vi "Climber_Sequencer.vi"() -> (0 "Outer_Arm_Elevator":dbl, 1 "Inner_Arm_Pivot":dbl, 2 "Outer_Arm_Pivot":dbl)   [LabVIEW 2020]
panel:
  in  "Inner_Arm_Pivot_No_Load":T1={"Kp"=0.1, "Ki"=0.1, "Kd"=0.1, "N-Diff"=10, "N-Int"=20, "Int Error Window"=0.5, "Max Ouput"=1.0, "Min Output"=-1.0} {"Int Error Window" min=0.0; "N-Int" min=2; "N-Diff" min=2; "Kd" min=0.0; "Ki" min=0.0; "Kp" min=0.0}
  in  "Outer_Arm_Pivot_On_Bar":T1={"Kp"=0.1, "Ki"=0.1, "Kd"=0.1, "N-Diff"=10, "N-Int"=20, "Int Error Window"=0.5, "Max Ouput"=1.0, "Min Output"=-1.0} {"Int Error Window" min=0.0; "N-Int" min=2; "N-Diff" min=2; "Kd" min=0.0; "Ki" min=0.0; "Kp" min=0.0}
  in  "Outer_Arm_Pivot_No_Load":T1={"Kp"=0.1, "Ki"=0.1, "Kd"=0.1, "N-Diff"=10, "N-Int"=20, "Int Error Window"=0.5, "Max Ouput"=1.0, "Min Output"=-1.0} {"Int Error Window" min=0.0; "N-Int" min=2; "N-Diff" min=2; "Kd" min=0.0; "Ki" min=0.0; "Kp" min=0.0}
  in  "Outer_Elevator_No_Load":T1={"Kp"=0.1, "Ki"=0.1, "Kd"=0.1, "N-Diff"=10, "N-Int"=20, "Int Error Window"=0.5, "Max Ouput"=1.0, "Min Output"=-1.0} {"Int Error Window" min=0.0; "N-Int" min=2; "N-Diff" min=2; "Kd" min=0.0; "Ki" min=0.0; "Kp" min=0.0}
  in  "Outer_Elevator_On_Bar":T1={"Kp"=0.1, "Ki"=0.1, "Kd"=0.1, "N-Diff"=10, "N-Int"=20, "Int Error Window"=0.5, "Max Ouput"=1.0, "Min Output"=-1.0} {"Int Error Window" min=0.0; "N-Int" min=2; "N-Diff" min=2; "Kd" min=0.0; "Ki" min=0.0; "Kp" min=0.0}
  in  "No PID":T1={"Kp"=0.1, "Ki"=0.1, "Kd"=0.1, "N-Diff"=10, "N-Int"=20, "Int Error Window"=0.5, "Max Ouput"=1.0, "Min Output"=-1.0} {"Int Error Window" min=0.0; "N-Int" min=2; "N-Diff" min=2; "Kd" min=0.0; "Ki" min=0.0; "Kp" min=0.0}
  in  "step 7 phi0 error leniency":dbl
  in  "d4":dbl
  in  "phi2 error leniency":dbl
  in  "phi2":dbl
  in  "d3":dbl
  in  "phi1 error leniency":dbl
  in  "phi1":dbl
  in  "d2":dbl
  in  "phi0":dbl=90.0 format="%#_13g"
  in  "theta1":dbl
  in  "theta0":dbl
  in  "move step back":bool
  in  "confirm step advance":bool
  in  "reset":bool
  in  "inner_arm_rotation":dbl
  in  "outer_arm_rotation":dbl
  in  "d1":dbl
  in  "outer_arm_position":dbl
  out "step":i32
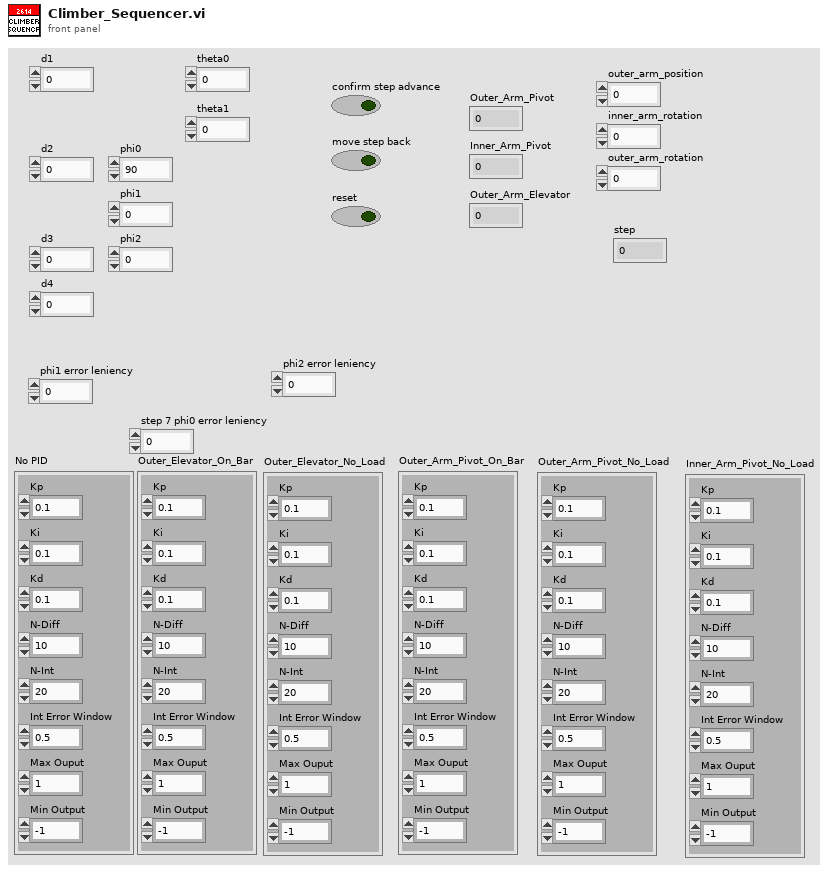
[diagram p1: front panel]
types:
  T1 = cluster{"Kp":dbl, "Ki":dbl, "Kd":dbl, "N-Diff":i32, "N-Int":i32, "Int Error Window":dbl, "Max Ouput":dbl, "Min Output":dbl}
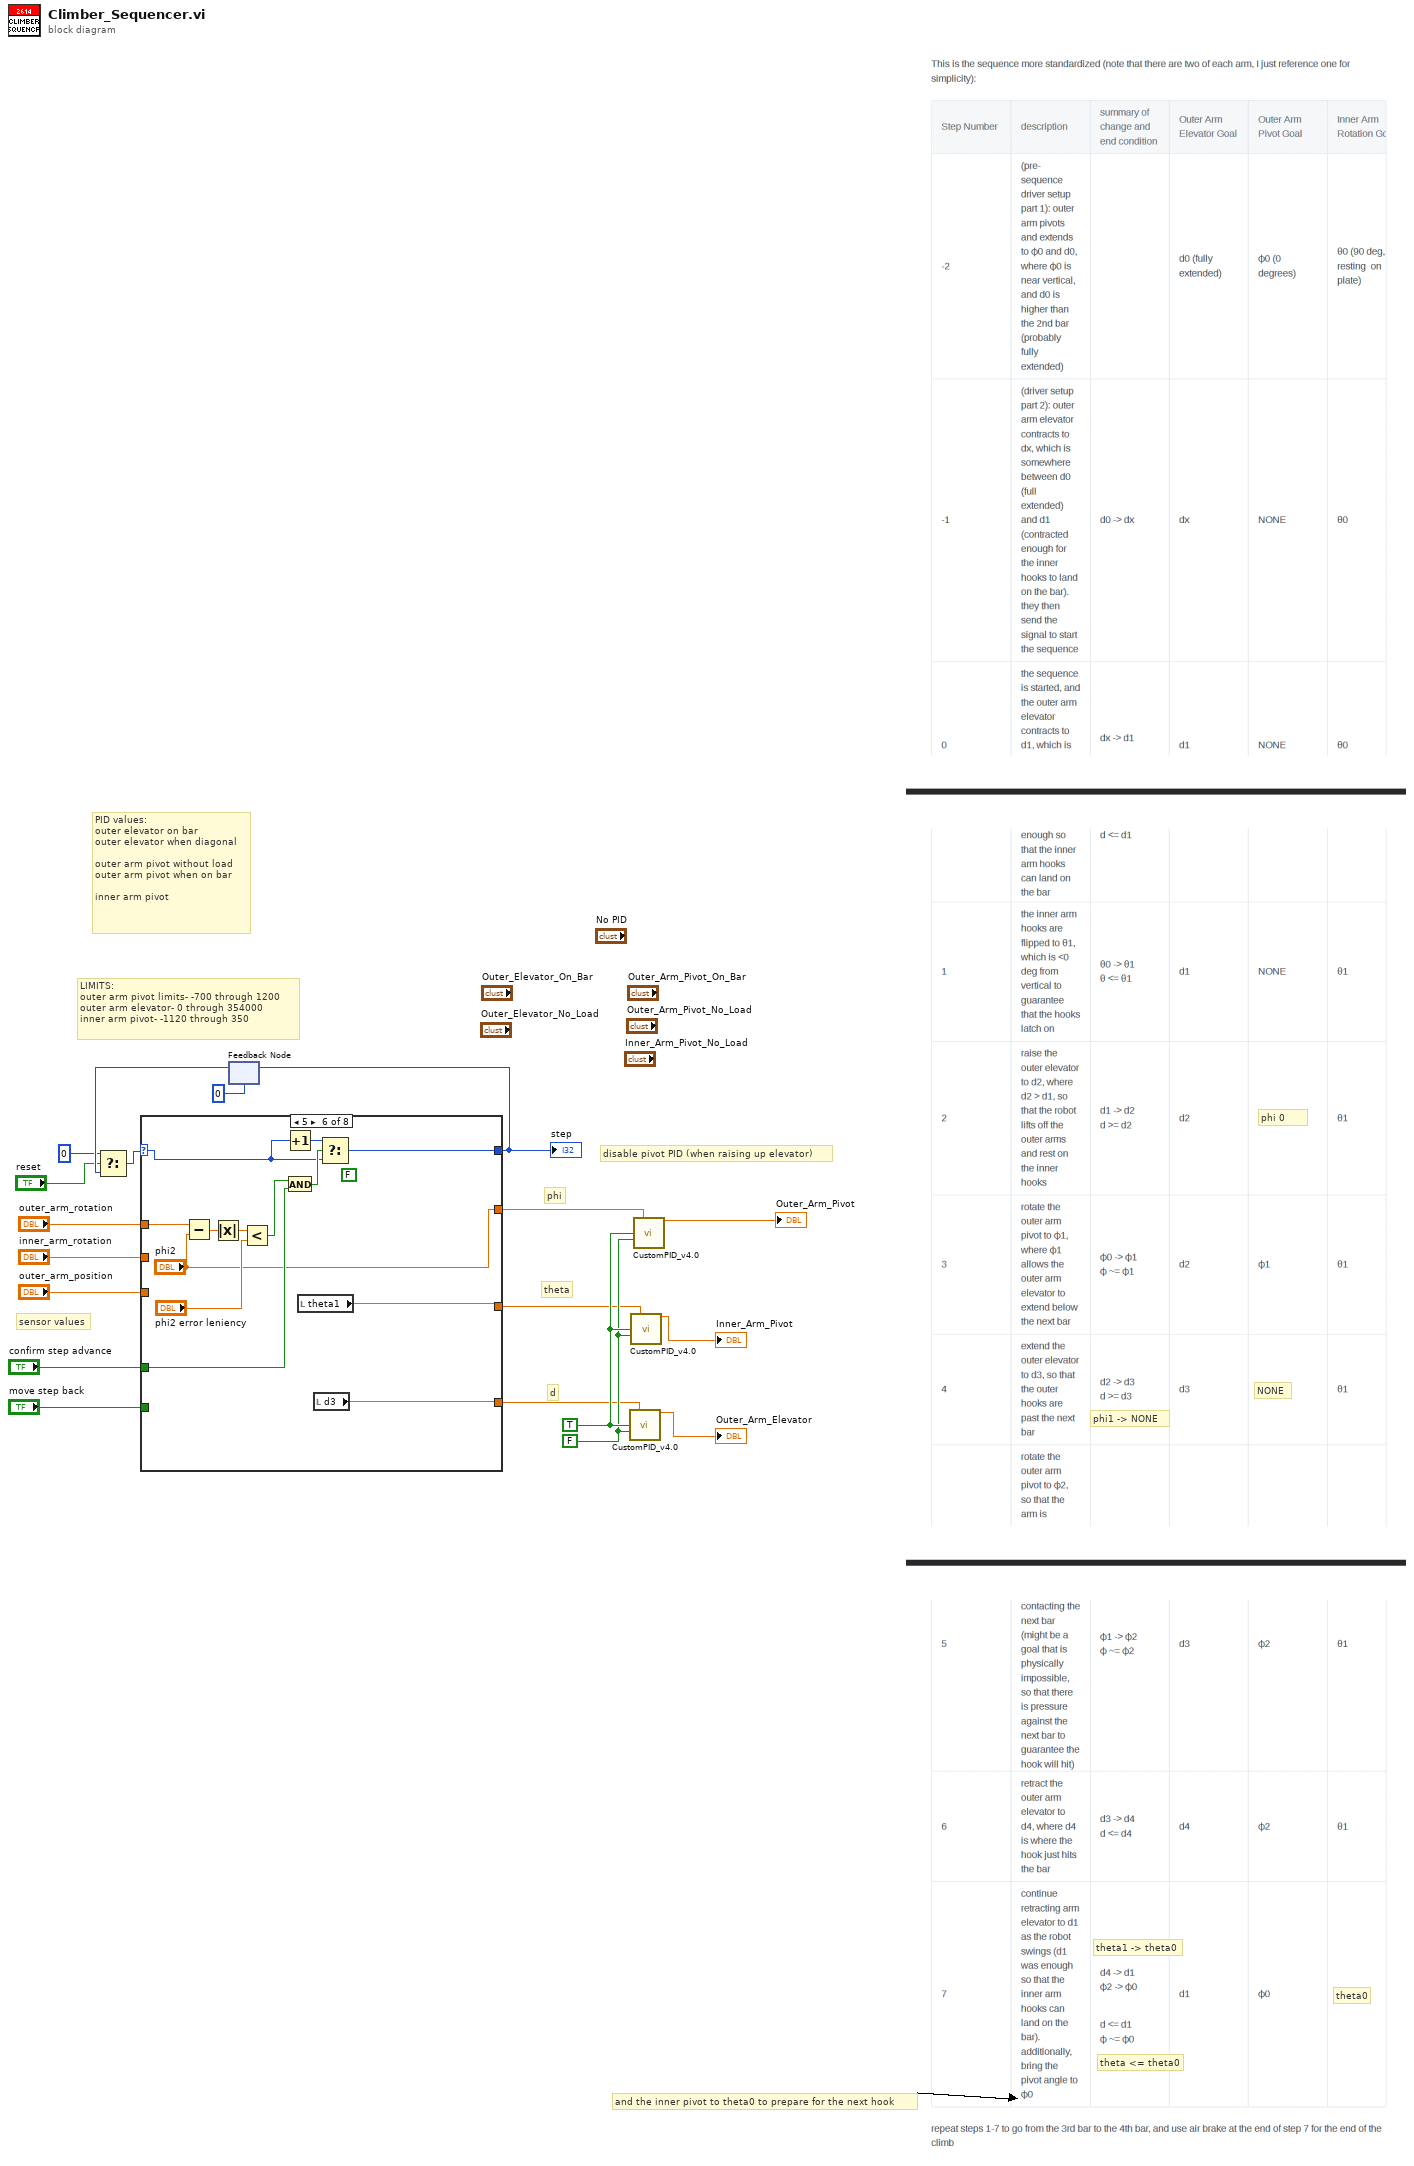
[diagram p0: block diagram]
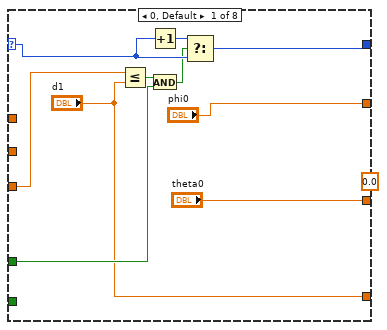
[diagram p2: hidden frame]
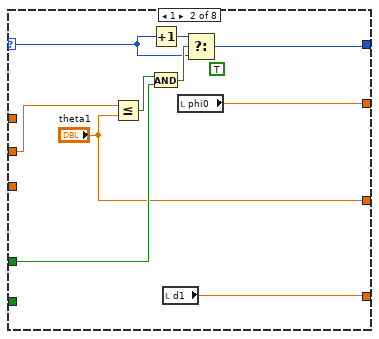
[diagram p3: hidden frame]
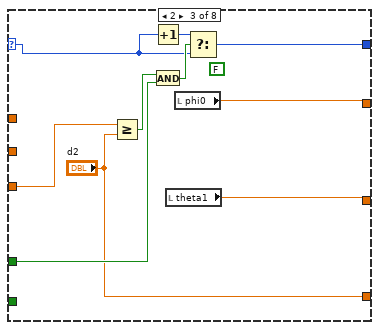
[diagram p4: hidden frame]
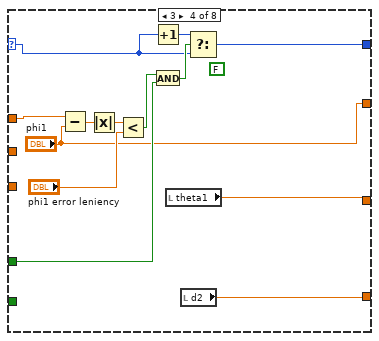
[diagram p5: hidden frame]
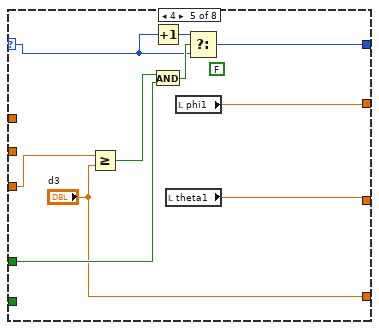
[diagram p6: hidden frame]
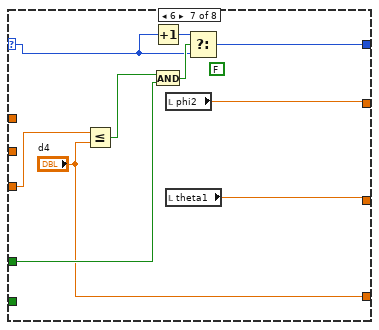
[diagram p7: hidden frame]
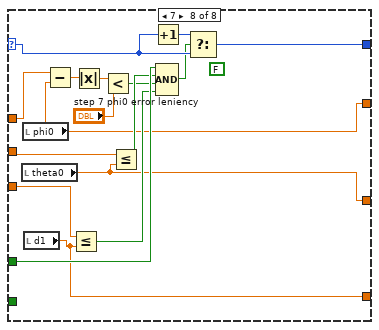
[diagram p8: hidden frame]
diagram:
  w9 = FALSE ("Reset on Goal Change ?")
  w10 = TRUE ("Reset on Goal Change ?")
  # "PID values:\nouter elevator on bar\nouter elevator when diagonal\n\nouter arm pivot without load\nouter arm pivot when on bar\n\ninner arm pivot"
  # "LIMITS:\nouter arm pivot limits- -700 through 1200\nouter arm elevator- 0 through 354000\ninner arm pivot- -1120 through 350"
  # "NONE"
  # "phi1 -> NONE"
  # "theta0"
  # "theta <= theta0"
  # "theta1 -> theta0"
  # "and the inner pivot to theta0 to prepare for the next hook"
  # "phi 0"
  # "disable pivot PID (when raising up elevator)"
  # "theta"
  # "phi"
  # "d"
  # "sensor values"
  n1 = feedback #1(0) -> (w16:i32)
  n2 = Select(t=0, s="reset", f=w16) -> (s? t:f=w17:i32)
  n3 = case shown="5" w17 {
    selector: w17 -> [w28 w36 w47 w60 w70 w83 w93 w111]
    tunnel: [w29 w37 w46 w59 w69 w82 w92 w110] -> w19
    tunnel: "outer_arm_position" -> [w26 _ w42 _ w65 _ w88 w107]
    tunnel: "confirm step advance" -> [w23 w35 w45 w58 w68 w81 w91 w108]
    tunnel: "move step back" -> [_ _ _ _ _ _ _ _]
    tunnel: ["phi0" w30 w44 "phi1" w66 "phi2" w89 w96] -> w6
    tunnel: "outer_arm_rotation" -> [_ _ _ w55 _ w77 _ w101]
    tunnel: "inner_arm_rotation" -> [_ w34 _ _ _ _ _ w103]
    tunnel: ["theta0" "theta1" w43 w57 w67 w80 w90 w102] -> w3
    tunnel: ["d1" w31 "d2" w56 "d3" w74 "d4" w105] -> w2
    frame 0, Default {
      (unwired) 0.0 ("d1")
      (unwired) 0.0 ("d1")
      n4 = Less Or Equal?(x=w26, y="d1") -> (x <= y?=w25:bool)
      n5 = Increment(x=w28) -> (x+1=w27:i32)
      n6 = And(x=w25, y=w23) -> (x .and. y?=w24:bool)
      n7 = Select(t=w27, s=w24, f=w28) -> (s? t:f=w29:i32)
    }
    frame 1 {
      (unwired) TRUE
      n8 = Less Or Equal?(x=w34, y="theta1") -> (x <= y?=w33:bool)
      n9 = Increment(x=w36) -> (x+1=w39:i32)
      n10 = And(x=w33, y=w35) -> (x .and. y?=w38:bool)
      n11 = local read "d1"() -> (w31:dbl)
      n12 = local read "phi0"() -> (w30:dbl)
      n13 = Select(t=w39, s=w38, f=w36) -> (s? t:f=w37:i32)
    }
    frame 2 {
      (unwired) FALSE
      n14 = Greater Or Equal?(x=w42, y="d2") -> (x >= y?=w41:bool)
      n15 = Increment(x=w47) -> (x+1=w49:i32)
      n16 = And(x=w41, y=w45) -> (x .and. y?=w48:bool)
      n17 = local read "theta1"() -> (w43:dbl)
      n18 = local read "phi0"() -> (w44:dbl)
      n19 = Select(t=w49, s=w48, f=w47) -> (s? t:f=w46:i32)
    }
    frame 3 {
      (unwired) FALSE
      n20 = Subtract(x=w55, y="phi1") -> (x-y=w54:dbl)
      n21 = Absolute Value(x=w54) -> (abs(x)=w53:dbl)
      n22 = Less?(x=w53, y="phi1 error leniency") -> (x < y?=w51:bool)
      n23 = Increment(x=w60) -> (x+1=w62:i32)
      n24 = And(x=w51, y=w58) -> (x .and. y?=w61:bool)
      n25 = local read "theta1"() -> (w57:dbl)
      n26 = local read "d2"() -> (w56:dbl)
      n27 = Select(t=w62, s=w61, f=w60) -> (s? t:f=w59:i32)
    }
    frame 4 {
      (unwired) FALSE
      n28 = Greater Or Equal?(x=w65, y="d3") -> (x >= y?=w64:bool)
      n29 = Increment(x=w70) -> (x+1=w72:i32)
      n30 = And(x=w64, y=w68) -> (x .and. y?=w71:bool)
      n31 = local read "theta1"() -> (w67:dbl)
      n32 = local read "phi1"() -> (w66:dbl)
      n33 = Select(t=w72, s=w71, f=w70) -> (s? t:f=w69:i32)
    }
    frame 5 {
      (unwired) FALSE
      n34 = Subtract(x=w77, y="phi2") -> (x-y=w79:dbl)
      n35 = Absolute Value(x=w79) -> (abs(x)=w78:dbl)
      n36 = Less?(x=w78, y="phi2 error leniency") -> (x < y?=w75:bool)
      n37 = Increment(x=w83) -> (x+1=w85:i32)
      n38 = And(x=w75, y=w81) -> (x .and. y?=w84:bool)
      n39 = local read "theta1"() -> (w80:dbl)
      n40 = local read "d3"() -> (w74:dbl)
      n41 = Select(t=w85, s=w84, f=w83) -> (s? t:f=w82:i32)
    }
    frame 6 {
      (unwired) FALSE
      n42 = Less Or Equal?(x=w88, y="d4") -> (x <= y?=w87:bool)
      n43 = Increment(x=w93) -> (x+1=w95:i32)
      n44 = And(x=w87, y=w91) -> (x .and. y?=w94:bool)
      n45 = local read "phi2"() -> (w89:dbl)
      n46 = local read "theta1"() -> (w90:dbl)
      n47 = Select(t=w95, s=w94, f=w93) -> (s? t:f=w92:i32)
    }
    frame 7 {
      (unwired) FALSE
      n48 = local read "theta0"() -> (w102:dbl)
      n49 = local read "phi0"() -> (w96:dbl)
      n50 = local read "d1"() -> (w105:dbl)
      n51 = Subtract(x=w101, y=w96) -> (x-y=w100:dbl)
      n52 = Less Or Equal?(x=w107, y=w105) -> (x <= y?=w106:bool)
      n53 = Absolute Value(x=w100) -> (abs(x)=w99:dbl)
      n54 = Less?(x=w99, y="step 7 phi0 error leniency") -> (x < y?=w97:bool)
      n55 = Less Or Equal?(x=w103, y=w102) -> (x <= y?=w104:bool)
      n56 = Increment(x=w111) -> (x+1=w112:i32)
      n57 = Compound Arithmetic op=AND(w108, w104, w97, w106) -> (w109:bool)
      n58 = Select(t=w112, s=w109, f=w111) -> (s? t:f=w110:i32)
    }
  }
  "step" <- w19
  n59 = feedback-in #1(w19) -> ()
  n60 = call "CustomPID_v4.0.vi"("Goal"=w2, "Reset on Goal Change ?"=w10, "Use Custom Error Calculation ?"=w9) -> ("Command"=→"Outer_Arm_Elevator":dbl)  [unwired: 9 in, 3 out]
  n61 = call "CustomPID_v4.0.vi"("Goal"=w3, "Reset on Goal Change ?"=w10, "Use Custom Error Calculation ?"=w9) -> ("Command"=→"Inner_Arm_Pivot":dbl)  [unwired: 9 in, 3 out]
  n62 = call "CustomPID_v4.0.vi"("Goal"=w6, "Reset on Goal Change ?"=w10, "Use Custom Error Calculation ?"=w9) -> ("Command"=→"Outer_Arm_Pivot":dbl)  [unwired: 9 in, 3 out]
